vi "DB Tools Fetch Table Data.vi"(4 "error in (no error)":errorcluster, 7 "recordset reference":T1) -> (0 "error out":errorcluster, 1 "recordset data":string[][](array[string]), 3 "recordset reference out":T1)   [LabVIEW 2020, in "NI_Database_API.lvlib"]
doc: "Returns all the <B>recordset data</B> referenced by <B>recordset reference</B> in the database as a 2D array of strings ( also a table data type in LabVIEW). This subVI has been optimized for performance."
uses:
  <vilib>/addons/database/NI_Database_API.lvlib
  <vilib>/addons/database/Recordset.llb/Rec ObjectReference.ctl
  <vilib>/addons/database/_DB Variant To Data/Database Variant To Data.xnode
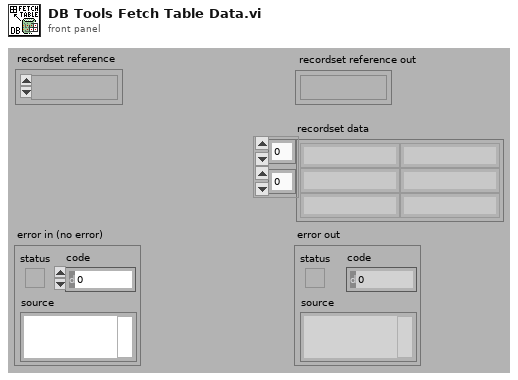
[diagram p1: front panel]
types:
  T1 = typedef "NI_Database_API.lvlib/Rec ObjectReference.ctl" = refnum<k1>
  T2 = typedef "NI_Database_API.lvlib/Rec DataMembers.ctl" = cluster{"ADODB._Recordset":refnum<k7>, "Connection":T3}
  T3 = typedef "NI_Database_API.lvlib/Conn ObjectReference.ctl" = refnum<k1>
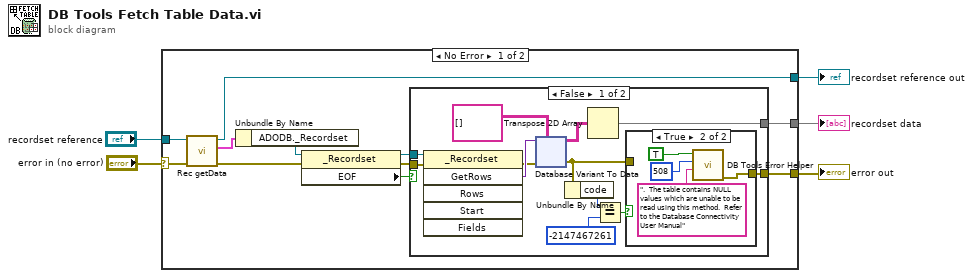
[diagram p0: block diagram]
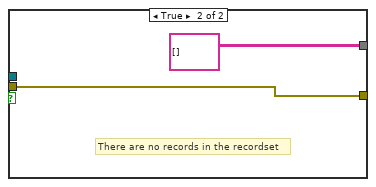
[diagram p3: hidden frame]
diagram:
  n1 = case shown="No Error" "error in (no error)" {
    selector: "error in (no error)" -> [w6 w69]
    tunnel: [w15 w69] -> w5
    tunnel: [w14 _] -> w4
    tunnel: "recordset reference" -> [w13 w68]
    tunnel: [w12 w68] -> w2
    frame No Error {
      n2 = call <vilib>:"Rec getData.vi"("error in (no error)"=w6, "recordset reference"=w13) -> ("error out"=w8:errorcluster, "data"=w16:T2, "recordset reference out"=w12:T1)  [unwired: 3 out]
      n3 = Unbundle By Name(w16) -> ("ADODB._Recordset"=w11:refnum<k7>)
      n4 = property class="_Recordset"(reference=w11, error in=w8) -> (reference out=w10:refnum<k7>, error out=w9:errorcluster, "EOF"=w7:bool)
      n5 = case shown="False" w7 {
        tunnel: [w22 w66] -> w15
        tunnel: [w27 string[][] [] ("recordset data")] -> w14
        tunnel: w9 -> [w26 w66]
        tunnel: w10 -> [w25 _]
        frame False {
          n6 = invoke class="_Recordset" method="GetRows"(reference=w25, error in=w26) -> (error out=w17:errorcluster, "GetRows"=w24:variant)  [unwired: 4 in, 4 out]
          n7 = xnode "Database Variant To Data"("database variant"=w24, "error in"=w17, "type"=string[][] [] ("recordset data")) -> ("data"=w28:string[][], "error out"=w21:errorcluster)
          n8 = Unbundle By Name(w21) -> ("code"=w20:i32)
          n9 = Transpose 2D Array(2D array=w28) -> (transposed array=w27:string[][])
          n10 = Equal?(x=w20, y=-2147467261) -> (x = y?=w19:bool)
          n11 = case shown="True" w19 {
            tunnel: w21 -> [w61 _]
            tunnel: [w61 w65] -> w22
            frame False {
            }
            frame True {
              n12 = call <vilib>:"DB Tools Error Helper.vi"("source"=".  The table contains NULL values which are unable to be read using this method.  Refer to the Database Connectivity User Manual", "code"=508, "status"=TRUE) -> ("error out"=w65:errorcluster)  [unwired: 1 in, 7 out]
            }
          }
        }
        frame True {
          # "There are no records in the recordset"
        }
      }
    }
    frame Error {
    }
  }
  "recordset reference out" <- w2
  "error out" <- w5
  "recordset data" <- w4
